vi "Main.vi"(11 "Module Admin":refnum<class "Delacor_lib_QMH_Module Admin.lvclass">) -> ()   [LabVIEW 2019, in "Notification.lvlib"]
doc: "This template is based off of the Queued Message Handler design pattern and the Queued Message Handler project template that ships with LabVIEW.\n\nThe main difference is that the queue is private to this module and communication between modules is performed via Broadcast and Request events.\n\nRequest events are wrapped in public API methods and are handled in the Event Handling Loop (EHL) of this VI. Any module can register for Broadcast events sent by this module. The EHL generates messages based on user interface actions.\n\nThe Message Handling Loop (MHL) processes messages generated by the EHL, or by other messages. The messages are string values, so new messages can be added easily to the Message Cases case structure in the MHL. Each message cluster can also provide an optional value for Message Data, which is a variant that can be converted to whatever message-specific data is required.\n_____\nBased on Delacor QMH Project Template 5.0.0.82."
uses:
  Notification.lvlib
  <vilib>/Delacor/Delacor QMH/Libraries/Module Admin_class/Delacor_lib_QMH_Module Admin.lvclass
  Module Data--cluster.ctl
  <vilib>/Delacor/Delacor QMH/Libraries/Message Queue_class/Delacor_lib_QMH_Message Queue.lvclass/Delacor_lib_QMH_Message Queue.ctl
  Stop Argument--cluster.ctl
  <vilib>/Delacor/Delacor QMH/Libraries/Module Admin_class/Delacor_lib_QMH_Module Admin.lvclass/Delacor_lib_QMH_Module Admin.ctl
  Send Telegram Argument--cluster.ctl
  <vilib>/Utility/miscctls.llb/LVPointTypeDef.ctl
  Telegram-Bot/Telegram/Methods/TypeDefs/SendMessageType.ctl
  <vilib>/Delacor/Delacor QMH/Libraries/Message Queue_class/Delacor_lib_QMH_Enqueue Message (Single).vi
  <vilib>/Delacor/Delacor QMH/Libraries/Module Admin_class/Delacor_lib_QMH_Get External Launch.vi
  <vilib>/Utility/error.llb/Error Cluster From Error Code.vi
  <vilib>/ErrorRing/Error Ring.xnode
  <vilib>/Delacor/Delacor QMH/Libraries/Message Queue_class/Delacor_lib_QMH_Message Queue.lvclass
  Camera/Camera.lvlib
panel:
  in  "Simulate MHL Error":bool
  in  "Simulate EHL Error":bool
  out "error out":errorcluster
  out "Status":string
  # "Other QMH Modules communicate with this Module via its Public API (wrappers for its Request Events).\n\nThis Module communicates with other Modules via its Broadcast Events.\nAny module that wants to get these messages, just registers for this module's Broadcast events."
  # "This template is for the Delacor Modified Queued Message Handler design pattern.\n\nSee the block diagram for more information on how to use this template."
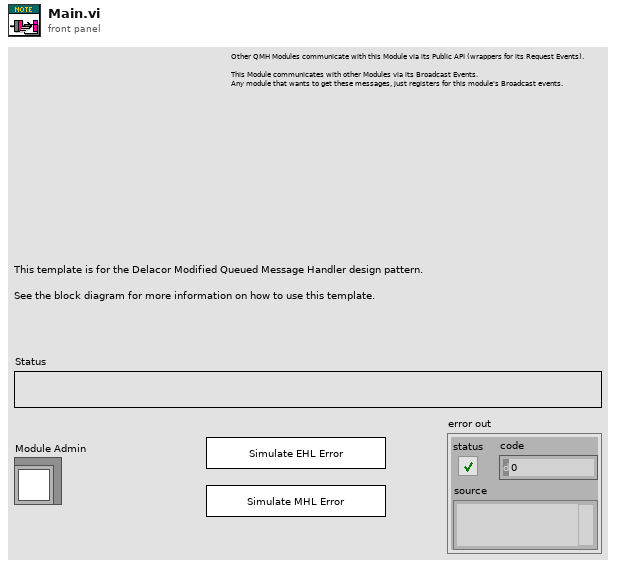
[diagram p1: front panel]
types:
  T1 = typedef "Notification.lvlib/Request Events--cluster.ctl" = cluster{"Stop Module":refnum<user-event>, "Show Panel":refnum<user-event>, "Hide Panel":refnum<user-event>, "Get Module Execution Status":refnum<user-event>, "Show Diagram":refnum<user-event>, "Send Telegram":refnum<user-event>}
  T2 = typedef "Camera.lvlib/Broadcast Events--cluster.ctl" = cluster{"Module Did Init":refnum<user-event>, "Status Updated":refnum<user-event>, "Error Reported":refnum<user-event>, "Module Did Stop":refnum<user-event>, "Update Module Execution Status":refnum<user-event>, "Broadcast Image":refnum<user-event>, "Broadcast Exposure Time":refnum<user-event>, "Broadcast Binning":refnum<user-event>, "Broadcast GatingMode":refnum<user-event>, "Broadcast RepetitiveGate":refnum<user-event>, "Broadcast IntensifierStatus":refnum<user-event>, "Broadcast IntensifierGain":refnum<user-event>, "Broadcast EMIccdGainControlMode":refnum<user-event>, "Broadcast EMIccdGain":refnum<user-event>, "Broadcast FloatingPoint Parameter":refnum<user-event>, "Broadcast Integer Parameter":refnum<user-event>}
  T3 = typedef "Notification.lvlib/Module Data--cluster.ctl" = cluster{"Status":string, "token":string, "chat_ids":cluster{"ntf_ids":i32[], "ntfcrit_ids":i32[]}}
  T4 = enum32{"invalid lock state", "Not Locked", "Locked (No Password)", "Password-protected"}
  T5 = typedef "Notification.lvlib/Stop Argument--cluster.ctl" = cluster{"Origin":string, "Exit via Stop Module Req?":bool, "Wait for Module to stop?":bool}
  T6 = typedef "Notification.lvlib/Send Telegram Argument--cluster.ctl" = cluster{"message":string}
  T7 = typedef "LVPointTypeDef.ctl" = cluster{"Horizontal":i16, "Vertical":i16}
  T8 = enum32{"Invalid", "Standard", "Closed", "Hidden", "Minimized", "Maximized"}
  T9 = typedef "SendMessageType.ctl" = enum16{"Text", "ReplyKeyboardMarkup", "ReplyKeyboardRemove"}
  T10 = typedef "UpdateUniversal.ctl" = cluster{"update_id":u32, "message":cluster{"message_id":u32, "from":cluster{"id":u64, "first_name":string}, "chat":cluster{"id":i32, "first_name":string, "type":string}, "date":u32, "text":string, "reply_to_message":cluster{"message_id":u32, "from":cluster{"id":u64, "first_name":string}, "chat":cluster{"id":i32, "first_name":string, "type":string}, "date":u32, "text":string}}}[]
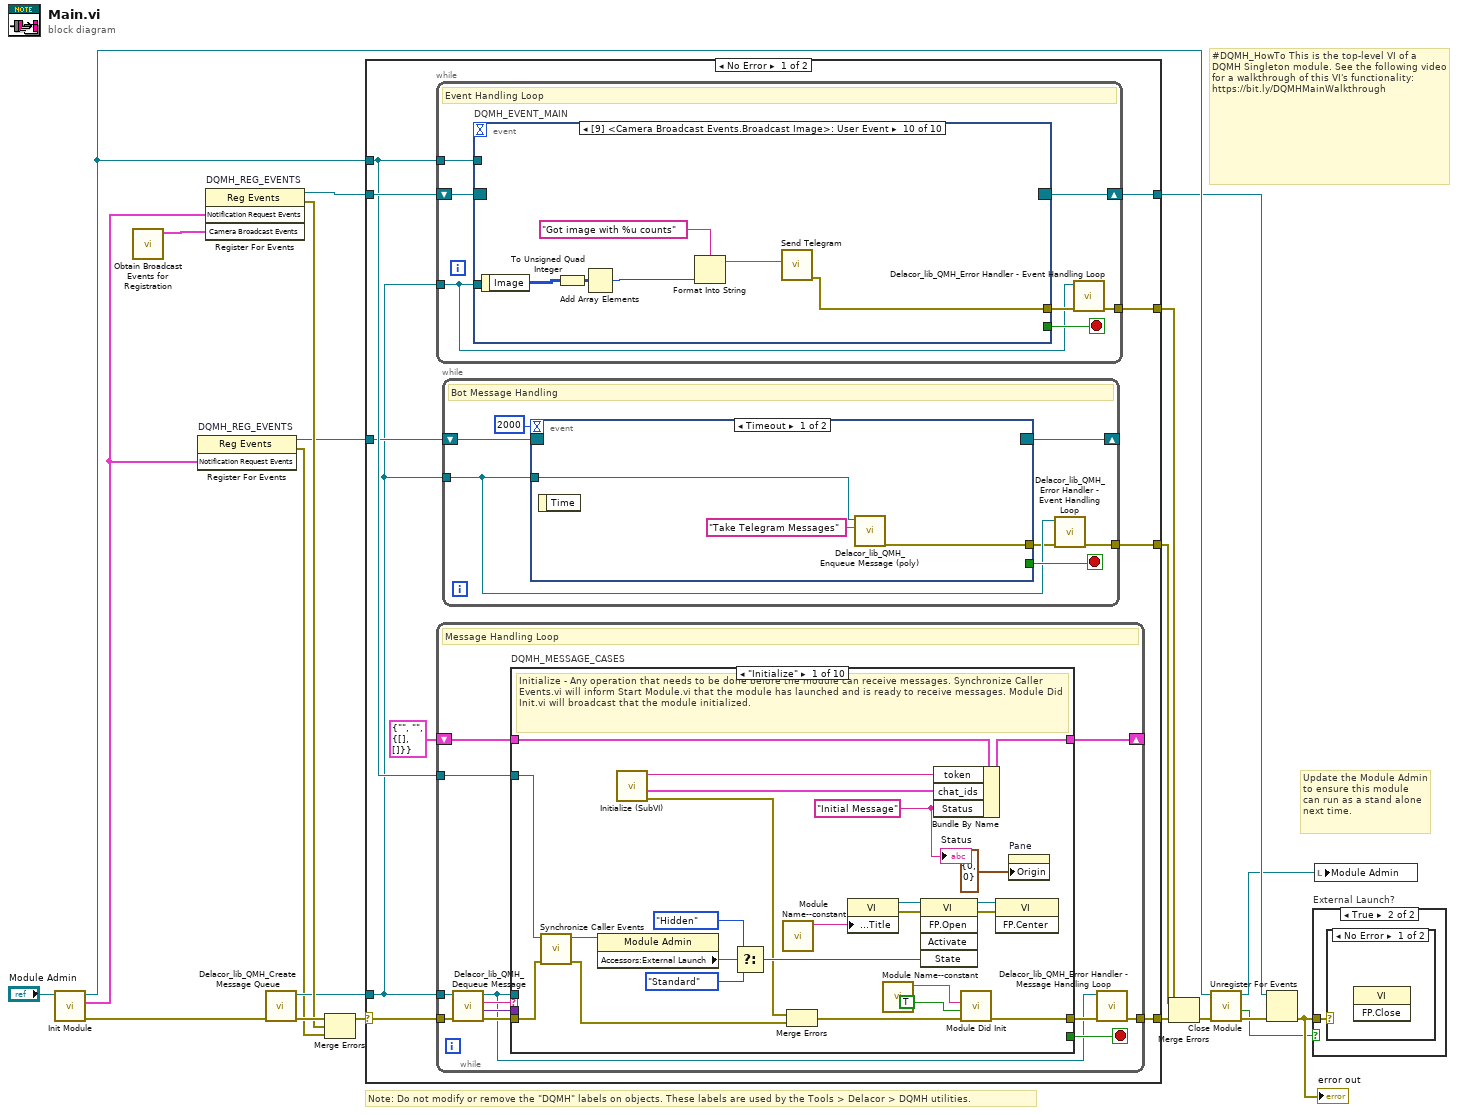
[diagram p0: block diagram]
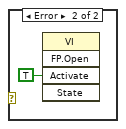
[diagram p3: hidden frame]
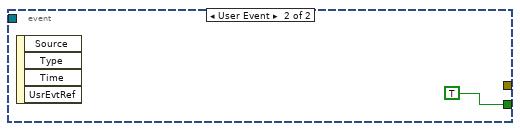
[diagram p4: hidden frame]
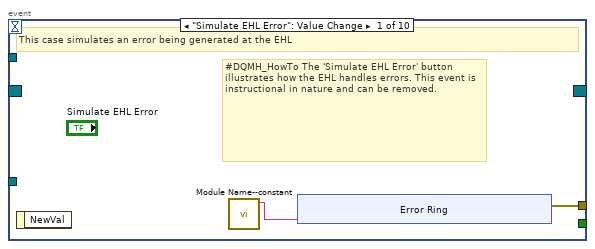
[diagram p5: hidden frame]
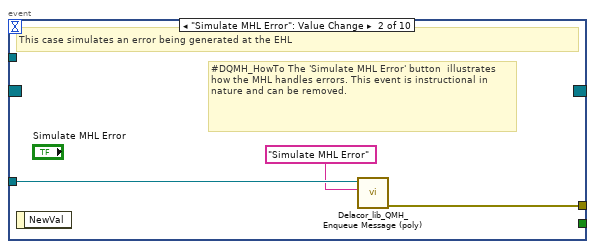
[diagram p6: hidden frame]
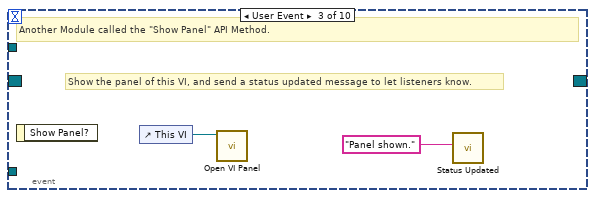
[diagram p7: hidden frame]
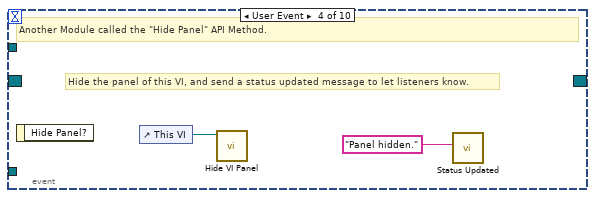
[diagram p8: hidden frame]
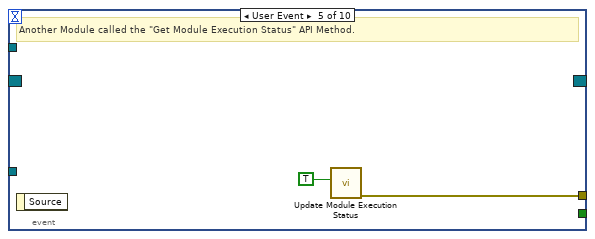
[diagram p9: hidden frame]
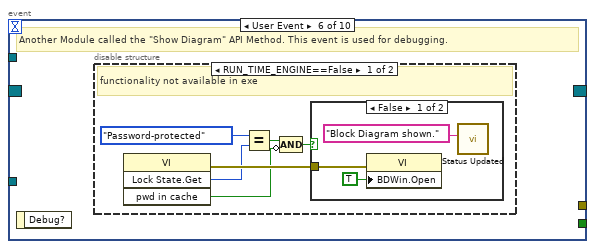
[diagram p10: hidden frame]
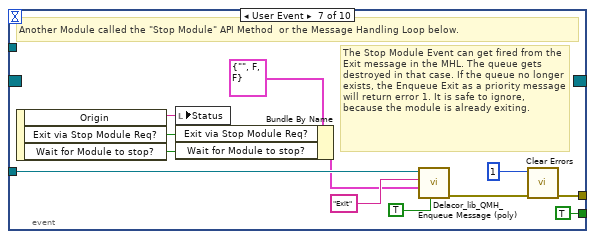
[diagram p13: hidden frame]
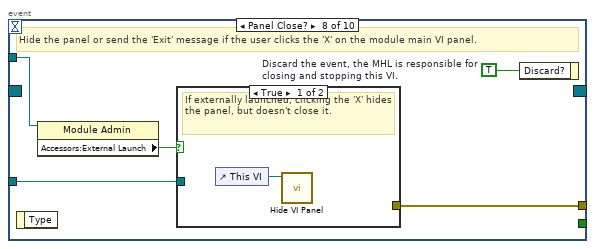
[diagram p14: hidden frame]
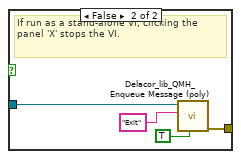
[diagram p15: hidden frame]
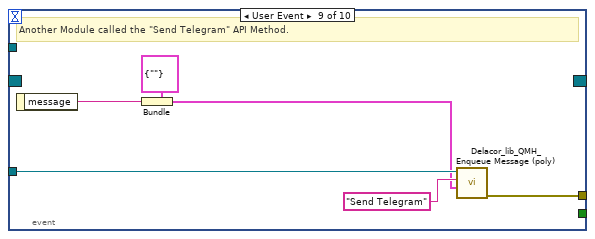
[diagram p16: hidden frame]
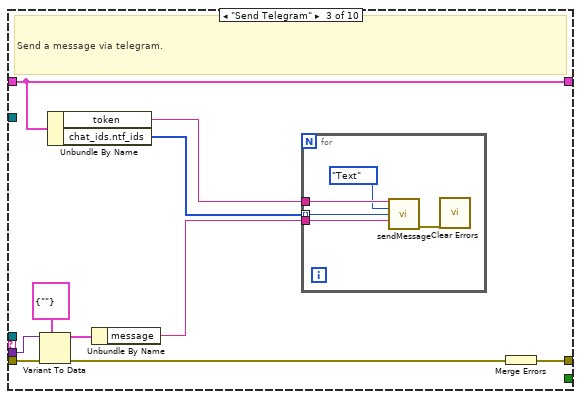
[diagram p18: hidden frame]
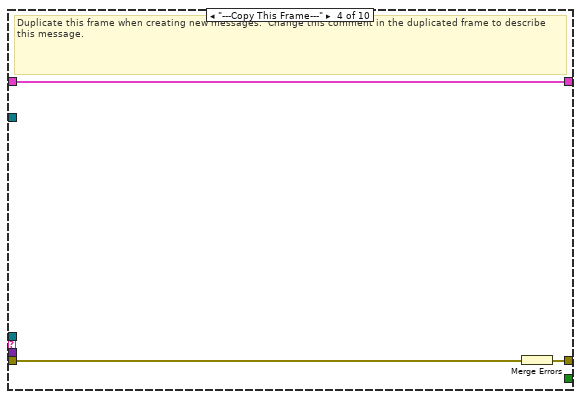
[diagram p19: hidden frame]
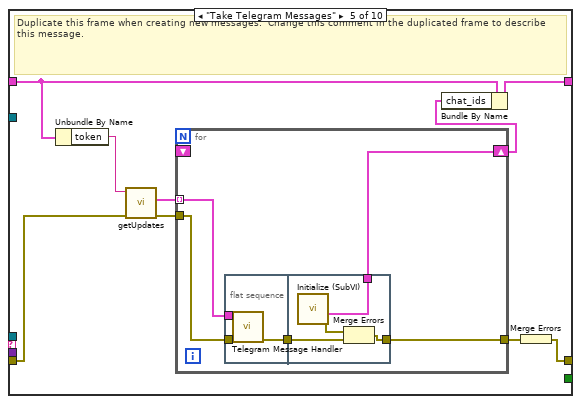
[diagram p20: hidden frame]
diagram:
  # "#DQMH_HowTo This is the top-level VI of a DQMH Singleton module. See the following video for a walkthrough of this VI's functionality: https://bit.ly/DQMHMainWalkthrough"
  # "Note: Do not modify or remove the \"DQMH\" labels on objects. These labels are used by the Tools > Delacor > DQMH utilities."
  # "Update the Module Admin to ensure this module can run as a stand alone next time."
  n1 = call "Init Module.vi"("Singleton Module Admin in"="Module Admin") -> ("error out"=w20:errorcluster, "Notification Request Events"=w5:T1, "Singleton Module Admin out"=w12:refnum<class "Delacor_lib_QMH_Module Admin.lvclass">)  [unwired: 8 in]
  n2 = call "Obtain Broadcast Events for Registration.vi"() -> ("Camera Broadcast Events"=w1:T2)  [unwired: 9 in, 2 out]
  n3 = register-events "DQMH_REG_EVENTS"(w5) -> (reference out=w3:refnum<event-registration>, error out=w4:errorcluster)  [unwired: 2 in]
  n4 = register-events "DQMH_REG_EVENTS"(w5, w1) -> (reference out=w10:refnum<event-registration>, error out=w13:errorcluster)  [unwired: 2 in]
  n5 = call <vilib>:"Delacor_lib_QMH_Create Message Queue.vi"("error in (no error)"=w20) -> ("error out"=w15:errorcluster, "Message Queue"=w9:refnum<class "Delacor_lib_QMH_Message Queue.lvclass">)  [unwired: 9 in]
  n6 = Merge Errors(w15, w13, w4) -> (w14:errorcluster)
  n7 = case shown="No Error" w14 {
    selector: w14 -> [w29 w250]
    tunnel: [w31 w249] -> w21
    tunnel: [w28 w255] -> w11
    tunnel: w10 -> [w26 w255]
    tunnel: w9 -> [w22 w248]
    tunnel: [w30 _] -> w18
    tunnel: w12 -> [w25 w251]
    tunnel: w3 -> [w24 _]
    tunnel: [w23 _] -> w2
    frame No Error {
      n8 = while {
        tunnel: w22 -> [w43]
        shift-right: [w46] -> w28
        shift-left: w26 -> [w47]
        tunnel: [w48] -> w30
        tunnel: w25 -> [w44]
        stop <- w45 stop-if-true
        # "Event Handling Loop"
        n9 = event "DQMH_EVENT_MAIN" shown="[9] <Camera Broadcast Events.Broadcast Image>: User Event" {
          selector: w47 -> [_ _ _ _ _ _ _ _ _ _]
          dyn-events: [_ _ _ _ _ _ _ _ _ _] -> w46
          timeout: _ -> [_ _ _ _ _ _ _ _ _ _]
          tunnel: [_ _ _ _ _ _ TRUE ("Discard?") _ _ _] -> w45
          tunnel: w43 -> [_ w60 _ _ _ _ w84 w91 w104 _]
          tunnel: [w51 w61 _ _ w67 _ w87 w93 w99 w105] -> w49
          tunnel: w44 -> [_ _ _ _ _ _ _ w90 _ _]
          event "Simulate EHL Error": Value Change {
            # "#DQMH_HowTo The 'Simulate EHL Error' button  illustrates how the EHL handles errors. This event is instructional in nature and can be removed."
            # "This case simulates an error being generated at the EHL"
            n10 = event-data() -> ()  [unwired: 1 in, 1 out]
            n11 = call "Module Name--constant.vi"() -> ("Module Name"=w50:string)  [unwired: 11 in]
            n12 = xnode "Error Ring"("parameter 0"=w50) -> ("error out"=w51:errorcluster)
          }
          event "Simulate MHL Error": Value Change {
            # "#DQMH_HowTo The 'Simulate MHL Error' button  illustrates how the MHL handles errors. This event is instructional in nature and can be removed."
            # "This case simulates an error being generated at the EHL"
            n13 = event-data() -> ()  [unwired: 1 in, 1 out]
            n14 = call-poly <vilib>:"Delacor_lib_QMH_Enqueue Message (poly).vi"("Message"="Simulate MHL Error", "Message Queue in"=w60) -> ("error out"=w61:errorcluster)  [unwired: 8 in, 1 out]
          }
          event User Event {
            # "Show the panel of this VI, and send a status updated message to let listeners know."
            # "Another Module called the \"Show Panel\" API Method."
            n15 = event-data() -> ()  [unwired: 1 in, 1 out]
            n16 = control-ref of="This VI"() -> (w63:refnum<vi>)
            n17 = call "Open VI Panel.vi"("VI"=w63) -> ()  [unwired: 10 in, 1 out]
            n18 = call "Status Updated.vi"("Status"="Panel shown." ("format string")) -> ()  [unwired: 10 in, 1 out]
          }
          event User Event {
            # "Hide the panel of this VI, and send a status updated message to let listeners know."
            # "Another Module called the \"Hide Panel\" API Method."
            n19 = event-data() -> ()  [unwired: 1 in, 1 out]
            n20 = control-ref of="This VI"() -> (w65:refnum<vi>)
            n21 = call "Hide VI Panel.vi"("VI"=w65) -> ()  [unwired: 10 in, 1 out]
            n22 = call "Status Updated.vi"("Status"="Panel hidden." ("format string")) -> ()  [unwired: 10 in, 1 out]
          }
          event User Event {
            # "Another Module called the \"Get Module Execution Status\" API Method."
            n23 = event-data() -> ()  [unwired: 1 in, 1 out]
            n24 = call "Update Module Execution Status.vi"("Running?"=TRUE) -> ("error out"=w67:errorcluster)  [unwired: 10 in]
          }
          event User Event {
            # "Another Module called the \"Show Diagram\" API Method. This event is used for debugging."
            n25 = event-data() -> ()  [unwired: 1 in, 1 out]
            n26 = disable-structure shown="RUN_TIME_ENGINE==False" {
              frame condition #0 (active) {
                # "functionality not available in exe"
                n27 = invoke class="VI" method="Lock State.Get"() -> (error out=w73:errorcluster, "Get Lock State"=w72:T4, "pwd in cache"=w69:bool)  [unwired: 4 in, 1 out]
                n28 = Equal?(x=T4."Password-protected", y=w72) -> (x = y?=w70:bool)
                n29 = Compound Arithmetic op=AND(w70, invert w69) -> (w68:bool)
                n30 = case shown="False" w68 {
                  tunnel: w73 -> [w76 _]
                  frame False {
                    n31 = property class="VI"(error in=w76, "BDWin.Open"=TRUE ("Block Diagram Window:Open")) -> ()  [unwired: 1 in, 2 out]
                    n32 = call "Status Updated.vi"("Status"="Block Diagram shown." ("format string")) -> ()  [unwired: 10 in, 1 out]
                  }
                  frame True {
                    # "Password-protected VI, and the password is not in the cache. Do not show the diagram."
                  }
                }
              }
              frame condition #1 {
              }
            }
          }
          event User Event {
            # "The Stop Module Event can get fired from the Exit message in the MHL. The queue gets destroyed in that case. If the queue no longer exists, the Enqueue Exit as a priority message will return error 1. It is safe to ignore, because the module is already exiting."
            # "Another Module called the \"Stop Module\" API Method  or the Message Handling Loop below."
            n33 = event-data() -> ("Origin"=w83:string, "Exit via Stop Module Req?"=w79:bool, "Wait for Module to stop?"=w78:bool)  [unwired: 1 in]
            n34 = local write "Status"(w83) -> ()
            n35 = Bundle By Name(cluster=T5 {"Origin"="", "Exit via Stop Module Req?"=FALSE, "Wait for Module to stop?"=FALSE} ("Stop Argument"), "Exit via Stop Module Req?"=w79, "Wait for Module to stop?"=w78) -> (w77:T5)
            n36 = call-poly <vilib>:"Delacor_lib_QMH_Enqueue Message (poly).vi"("Priority Message? (F)"=TRUE, "Message Data"=w77, "Message"="Exit", "Message Queue in"=w84) -> ("error out"=w88:errorcluster)  [unwired: 6 in, 1 out]
            n37 = call <vilib>:"Clear Errors.vi"("error in (no error)"=w88, "specific error code to clear (0: all)"=1) -> ("error out"=w87:errorcluster)  [unwired: 4 in, 1 out]
          }
          event Panel Close? {
            w92 = TRUE  # Discard the event, the MHL is responsible for closing and stopping this VI.
            # "Hide the panel or send the 'Exit' message if the user clicks the 'X' on the module main VI panel."
            n38 = event-data() -> ()  [unwired: 1 in, 1 out]
            n39 = property class="Module Admin"(reference=w90) -> ("Accessors:External Launch"=w89:bool)  [unwired: 1 in, 2 out]
            n40 = case shown="True" w89 {
              tunnel: w91 -> [_ w97]
              tunnel: [_ w98] -> w93
              frame True {
                # "If externally launched, clicking the 'X' hides the panel, but doesn't close it."
                n41 = control-ref of="This VI"() -> (w94:refnum<vi>)
                n42 = call "Hide VI Panel.vi"("VI"=w94) -> ()  [unwired: 10 in, 1 out]
              }
              frame False {
                # "If run as a stand-alone VI, clicking the panel 'X' stops the VI."
                n43 = call-poly <vilib>:"Delacor_lib_QMH_Enqueue Message (poly).vi"("Priority Message? (F)"=TRUE, "Message"="Exit", "Message Queue in"=w97) -> ("error out"=w98:errorcluster)  [unwired: 7 in, 1 out]
              }
            }
            n44 = event-data("Discard?"=w92) -> ()  [unwired: 1 in, 1 out]
          }
          event User Event {
            # "Another Module called the \"Send Telegram\" API Method."
            n45 = event-data() -> ("message"=w100:string)  [unwired: 1 in]
            n46 = Bundle(cluster=T6 {"message"=""} ("Send Telegram Argument"), "message"=w100) -> (w101:T6)
            n47 = call-poly <vilib>:"Delacor_lib_QMH_Enqueue Message (poly).vi"("Message Data"=w101, "Message"="Send Telegram", "Message Queue in"=w104) -> ("error out"=w99:errorcluster)  [unwired: 7 in, 1 out]
          }
          event User Event {
            n48 = event-data() -> ("Image"=w110:u16[][])  [unwired: 1 in]
            n49 = To Unsigned Quad Integer(1:w110) -> (0:w108:u64[][])
            n50 = Add Array Elements(numeric array=w108) -> (sum=w109:u64)
            n51 = Format Into String(format string="Got image with %u counts", w109) -> (resulting string=w106:string)  [unwired: 2 in, 1 out]
            n52 = call "Send Telegram.vi"("message"=w106) -> ("error out"=w105:errorcluster)  [unwired: 9 in]
          }
        }
        n53 = call-dynamic "Delacor_lib_QMH_Error Handler - Event Handling Loop.vi"("error in (no error)"=w49, "Message Queue in"=w43) -> ("dup error in"=w48:errorcluster)  [unwired: 8 in, 1 out]
      }
      n54 = while {
        tunnel: w22 -> [w113]
        shift-right: [w117] -> _
        shift-left: T3 {"Status"="", "token"="", "chat_ids"={"ntf_ids"=[], "ntfcrit_ids"=[]}} ("Data Cluster") -> [w118]
        tunnel: w29 -> [w121]
        tunnel: [w119] -> w31
        tunnel: w25 -> [w111]
        stop <- w116 stop-if-true
        # "Message Handling Loop"
        n55 = call-dynamic "Delacor_lib_QMH_Dequeue Message.vi"("error in (no error)"=w121, "Message Queue in"=w113) -> ("error out"=w120:errorcluster, "Message Data"=w114:variant, "Message"=w115:string, "Message Queue out"=w112:refnum<class "Delacor_lib_QMH_Message Queue.lvclass">)  [unwired: 6 in]
        n56 = case "DQMH_MESSAGE_CASES" shown="\"Initialize\"" w115 {
          selector: w115 -> [_ _ _ _ _ _ _ _ _ w235]
          tunnel: w112 -> [_ _ _ _ _ _ _ w205 w227 _]
          tunnel: w120 -> [w144 w148 w158 w166 w174 w189 w194 w212 w233 w237]
          tunnel: [w142 w148 w149 w165 w175 w189 w193 w208 w230 w238] -> w122
          tunnel: w118 -> [w133 w147 w153 w164 w170 w188 w191 w207 w226 w236]
          tunnel: [w132 w147 w153 w164 w168 w188 w191 w207 w226 w236] -> w117
          tunnel: [_ _ _ _ _ _ _ _ w225 _] -> w116
          tunnel: w114 -> [_ _ w156 _ _ _ _ w206 w224 _]
          tunnel: w111 -> [w134 _ _ _ _ _ _ w204 w219 _]
          frame "Initialize" {
            w127 = "Initial Message" ("Initial Message")
            # "Initialize - Any operation that needs to be done before the module can receive messages. Synchronize Caller Events.vi will inform Start Module.vi that the module has launched and is ready to receive messages. Module Did Init.vi will broadcast that the module initialized."
            n57 = call "Synchronize Caller Events.vi"("error in (no error)"=w144, "Singleton Module Admin in"=w134) -> ("error out"=w143:errorcluster, "Singleton Module Admin out"=w129:refnum<class "Delacor_lib_QMH_Module Admin.lvclass">)  [unwired: 8 in]
            n58 = property class="Module Admin"(reference=w129) -> ("Accessors:External Launch"=w138:bool)  [unwired: 1 in, 2 out]
            n59 = call "Initialize (SubVI).vi"() -> ("error out"=w124:errorcluster, "Cluster"=w123:cluster{"ntf_ids":i32[], "ntfcrit_ids":i32[]}, "token"=w126:string)  [unwired: 9 in]
            n60 = Select(t=T8."Hidden" ("State"), s=w138, f=T8."Standard" ("State")) -> (s? t:f=w135:T8)
            n61 = call "Module Name--constant.vi"() -> ("Module Name"=w141:string)  [unwired: 11 in]
            n62 = Merge Errors(w124, w143) -> (w125:errorcluster)
            n63 = property class="VI"("Front Panel.Title"=w141) -> (reference out=w140:refnum<vi>, error out=w146:errorcluster)  [unwired: 2 in]
            n64 = call "Module Name--constant.vi"() -> ("Module Name"=w130:string)  [unwired: 11 in]
            n65 = invoke class="VI" method="FP.Open"(reference=w140, error in=w146, "State"=w135) -> (reference out=w139:refnum<vi>, error out=w145:errorcluster)  [unwired: 2 in, 3 out]
            n66 = Bundle By Name(cluster=w133, "token"=w126, "chat_ids"=w123, "Status"=w127) -> (w132:T3)
            n67 = call "Module Did Init.vi"("error in (no error)"=w125, "Initialized?"=TRUE, "Origin"=w130) -> ("error out"=w142:errorcluster)  [unwired: 8 in]
            n68 = invoke class="VI" method="FP.Center"(reference=w139, error in=w145) -> ()  [unwired: 1 in, 3 out]
            n69 = property on="Pane" class="Pane"("Origin"=T7 {"Horizontal"=0, "Vertical"=0}) -> ()  [unwired: 2 in, 2 out]
            "Status" <- w127
          }
          frame "--- Module Specific ---" {
            # "Separator -- The following cases handle messages specific to this Module."
          }
          frame "Send Telegram" {
            # "Send a message via telegram."
            n70 = Variant To Data(error in=w158, type=T6 {"message"=""} ("Send Telegram Argument"), Variant=w156) -> (data=w154:T6, error out=w157:errorcluster)
            n71 = Unbundle By Name(w153) -> ("token"=w152:string, "chat_ids.ntf_ids"=w151:i32[])
            n72 = Unbundle By Name(w154) -> ("message"=w150:string)
            n73 = for {
              tunnel: w152 -> [w163]
              tunnel: w151 -> [w161] mode=indexing
              tunnel: w150 -> [w160]
              n74 = call "sendMessage.vi"("Token"=w163, "MsgType"=SendMessageType."Text", "ChatId"=w161, "Text"=w160) -> ("error out"=w159:errorcluster)  [unwired: 11 in]
              n75 = call <vilib>:"Clear Errors.vi"("error in (no error)"=w159) -> ()  [unwired: 5 in, 2 out]
            }
            n76 = Merge Errors(w157) -> (w149:errorcluster)
          }
          frame "---Copy This Frame---" {
            # "Duplicate this frame when creating new messages.  Change this comment in the duplicated frame to describe this message."
            n77 = Merge Errors(w166) -> (w165:errorcluster)
          }
          frame "Take Telegram Messages" {
            # "Duplicate this frame when creating new messages.  Change this comment in the duplicated frame to describe this message."
            n78 = Unbundle By Name(w170) -> ("token"=w169:string)
            n79 = call "getUpdates.vi"("error in"=w174, "Token"=w169) -> ("error out"=w172:errorcluster, "UpdateUniversal"=w171:T10)  [unwired: 6 in, 2 out]
            n80 = for {
              tunnel: [w178] -> w173
              tunnel: w172 -> [w180]
              tunnel: w171 -> [w179] mode=indexing
              shift-right: [w176] -> w167
              shift-left: _ -> [_]
              n81 = flat-sequence {
                tunnel: w180 -> [w183]
                tunnel: w179 -> [w182]
                tunnel: [w181] -> w177
                tunnel: [w187] -> w178
                tunnel: w177 -> [w186]
                tunnel: [w184] -> w176
                frame #0 {
                  n82 = call "Telegram Message Handler.vi"("error in (no error)"=w183, "Update"=w182) -> ("error out"=w181:errorcluster)  [unwired: 9 in]
                }
                frame #1 {
                  n83 = call "Initialize (SubVI).vi"() -> ("error out"=w185:errorcluster, "Cluster"=w184:cluster{"ntf_ids":i32[], "ntfcrit_ids":i32[]})  [unwired: 9 in, 1 out]
                  n84 = Merge Errors(w185, w186) -> (w187:errorcluster)
                }
              }
            }
            n85 = Bundle By Name(cluster=w170, "chat_ids"=w167) -> (w168:T3)
            n86 = Merge Errors(w173) -> (w175:errorcluster)
          }
          frame "--- Exit and Error Handling---" {
            # "Separator - The following cases handle errors and exit messages."
          }
          frame "Simulate MHL Error" {
            # "#DQMH_HowTo The 'Simulate MHL Error' button  illustrates how the MHL handles errors. This event is instructional in nature and can be removed."
            # "Simulate an error occurring at the MHL"
            n87 = call "Module Name--constant.vi"() -> ("Module Name"=w190:string)  [unwired: 11 in]
            n88 = xnode "Error Ring"("parameter 0"=w190) -> ("error out"=w192:errorcluster)
            n89 = Merge Errors(w194, w192) -> (w193:errorcluster)
          }
          frame "Error" {
            # "#CodeRecommended - If you ever change the name of this \"Error\" message, you'll need to update the name in the Check Loop Error.vi as well."
            # "#CodeRecommended - If the module is running in standalone mode (External Launch = FALSE), this code will pop up an error dialog and call the 'Exit' message if an error occurs. Add more fine-grained error handling here."
            # "Error - Check the error message data and respond accordingly. This message is sent by the \"Error Handler\" VIs at the end of each loop in this application."
            n90 = property class="Module Admin"(reference=w204) -> ("Accessors:External Launch"=w203:bool)  [unwired: 1 in, 2 out]
            n91 = Variant To Data(error in=w212, type=errorcluster {"status"=FALSE, "code"=0, "source"=""} ("error constant"), Variant=w206) -> (data=w213:errorcluster, error out=w210:errorcluster)
            n92 = call "Module Name--constant.vi"() -> ("Module Name"=w202:string)  [unwired: 11 in]
            n93 = call "Error Reported.vi"("Additional Information"=w202, "Error"=w213) -> ()  [unwired: 9 in, 1 out]
            n94 = case shown="False" w203 {
              tunnel: [w218 _] -> w209
              tunnel: w205 -> [w216 _]
              tunnel: w213 -> [w217 _]
              frame False {
                # "If the module is running standalone, then pop up an error dialog and call the \"Exit\" message."
                n95 = call <vilib>:"Simple Error Handler.vi"("error in (no error)"=w217) -> ()  [unwired: 4 in, 5 out]
                n96 = call-poly <vilib>:"Delacor_lib_QMH_Enqueue Message (poly).vi"("Priority Message? (F)"=TRUE, "Message"="Exit", "Message Queue in"=w216) -> ("error out"=w218:errorcluster)  [unwired: 7 in, 1 out]
              }
              frame True {
                # "If the module was launched externally, calling the Error Reported broadcast VI is the only action performed by the \"Error\" message. The module's caller can then process the error appropriately."
              }
            }
            n97 = Merge Errors(w210, w209) -> (w208:errorcluster)
            n98 = local write "error out"(w208) -> ()
          }
          frame "Exit" {
            w223 = 91  # 91: not all Exit messages will have an argument
            w225 = TRUE  # Stop the VI
            # "Release the message queue reference"
            # "#CodeNeeded - Add any required cleanup code here"
            # "Exit - Exit the application."
            n99 = Variant To Data(error in=w233, type=T5 {"Origin"="", "Exit via Stop Module Req?"=FALSE, "Wait for Module to stop?"=FALSE} ("Stop Argument"), Variant=w224) -> (data=w221:T5, error out=w229:errorcluster)
            n100 = call <vilib>:"Clear Errors.vi"("error in (no error)"=w229, "specific error code to clear (0: all)"=w223) -> ("error out"=w232:errorcluster)  [unwired: 4 in, 1 out]
            n101 = control-ref of="This VI"() -> (w220:refnum<vi>)
            n102 = call-dynamic "Delacor_lib_QMH_Release Message Queue.vi"("error in (no error)"=w232, "Message Queue"=w227) -> ("error out"=w231:errorcluster)  [unwired: 9 in]
            n103 = call "Handle Exit.vi"("Stop Argument"=w221, "Admin in"=w219, "VI reference"=w220) -> ("error out"=w228:errorcluster)  [unwired: 7 in, 1 out]
            n104 = Merge Errors(w231, w228) -> (w230:errorcluster)
          }
          frame Default {
            # "'Default' case only runs if there is a message that isn't defined in any of the other cases.  Output a programming error."
            n105 = call "Module Name--constant.vi"() -> ("Module Name"=w234:string)  [unwired: 11 in]
            n106 = xnode "Error Ring"("parameter 0"=w235, "parameter 1"=w234) -> ("error out"=w239:errorcluster)
            n107 = Merge Errors(w237, w239) -> (w238:errorcluster)
          }
        }
        n108 = call-dynamic "Delacor_lib_QMH_Error Handler - Message Handling Loop.vi"("error in (no error)"=w122, "Message Queue in"=w112) -> ("dup error in"=w119:errorcluster)  [unwired: 8 in, 1 out]
      }
      n109 = while {
        shift-right: [w35] -> _
        shift-left: w24 -> [w37]
        tunnel: [w34] -> w23
        tunnel: w22 -> [w33]
        stop <- w36 stop-if-true
        # "Bot Message Handling"
        n110 = event shown="[0] Timeout" {
          selector: w37 -> [_ _]
          dyn-events: [_ _] -> w35
          timeout: 2000 -> [_ _]
          tunnel: [_ TRUE] -> w36
          tunnel: w33 -> [w39 _]
          tunnel: [w41 _] -> w32
          event Timeout {
            n111 = event-data() -> ()  [unwired: 1 in, 1 out]
            n112 = call-poly <vilib>:"Delacor_lib_QMH_Enqueue Message (poly).vi"("Message"="Take Telegram Messages", "Message Queue in"=w39) -> ("error out"=w41:errorcluster)  [unwired: 8 in, 1 out]
          }
          event User Event {
            n113 = event-data() -> ()  [unwired: 1 in, 4 out]
          }
        }
        n114 = call-dynamic "Delacor_lib_QMH_Error Handler - Event Handling Loop.vi"("error in (no error)"=w32, "Message Queue in"=w33) -> ("dup error in"=w34:errorcluster)  [unwired: 8 in, 1 out]
      }
    }
    frame Error {
      # "Synchronize Caller Events.vi will inform Start Module.vi that the module has launched and will let the code calling Start Module.vi register for broadcasts and would permit the caller receive the broadcast that an error occurred at launch time."
      n115 = call-dynamic "Delacor_lib_QMH_Release Message Queue.vi"("error in (no error)"=w250, "Message Queue"=w248) -> ("error out"=w249:errorcluster)  [unwired: 9 in]
      n116 = call "Synchronize Caller Events.vi"("Singleton Module Admin in"=w251) -> ("error out"=w256:errorcluster)  [unwired: 9 in, 1 out]
      n117 = call "Module Name--constant.vi"() -> ("Module Name"=w254:string)  [unwired: 11 in]
      n118 = Format Into String(format string="An error occurred during initialization. %s is no longer running.", w254) -> (resulting string=w252:string)  [unwired: 2 in, 1 out]
      n119 = Merge Errors(w249, w256) -> (w257:errorcluster)
      n120 = call "Error Reported.vi"("Additional Information"=w252, "Error"=w257) -> ()  [unwired: 9 in, 1 out]
    }
  }
  n121 = Merge Errors(w2, w18, w21) -> (w17:errorcluster)
  n122 = call "Close Module.vi"("error in (no error)"=w17, "Module Admin in"=w12) -> ("error out"=w19:errorcluster, "External Launch"=w6:bool, "Module Admin out"=w7:refnum<class "Delacor_lib_QMH_Module Admin.lvclass">)  [unwired: 7 in]
  n123 = Unregister For Events(event registration refnum=w11, error in=w19) -> (error out=w16:errorcluster)
  "error out" <- w16
  n124 = case "External Launch?" shown="True" w6 {
    tunnel: w16 -> [_ w258]
    frame False {
    }
    frame True {
      n125 = case shown="No Error" w258 {
        frame No Error {
          n126 = invoke class="VI" method="FP.Close"() -> ()  [unwired: 3 in, 3 out]
        }
        frame Error {
          n127 = invoke class="VI" method="FP.Open"("Activate"=TRUE ("Activate?")) -> ()  [unwired: 4 in, 5 out]
        }
      }
    }
  }
  n128 = local write "Module Admin"(w7) -> ()
